vi "subsample_time_domain.vi"(8 "Array":cluster{"Array":dbl[]}[](array[cluster]), 10 "# sample points":i32, 11 "input array":dbl[][](array[numeric])) -> (3 "subsampled array":dbl[][](array[numeric]))   [LabVIEW 2016]
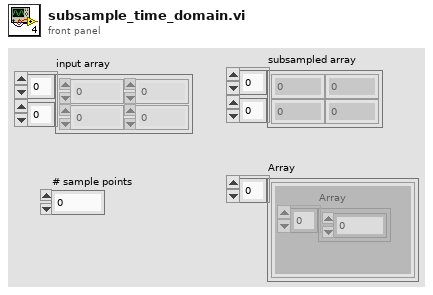
[diagram p1: front panel]
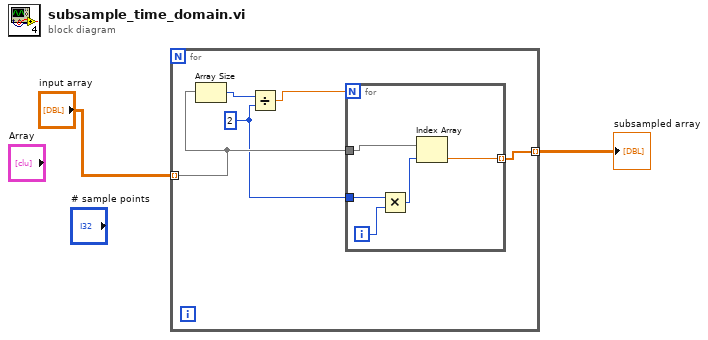
[diagram p0: block diagram]
diagram:
  n1 = for {
    tunnel: [w7] -> w2 mode=indexing
    tunnel: "input array" -> [w6] mode=indexing
    w3 = 2
    n2 = Array Size(array=w6) -> (size(s)=w5:i32)
    n3 = Divide(x=w5, y=w3) -> (x/y=w4:dbl)
    n4 = for {
      N: w4 -> [_]
      tunnel: w6 -> [w12]
      tunnel: [w10] -> w7 mode=indexing
      tunnel: w3 -> [w8]
      i -> [w9]
      n5 = Multiply(x=w8, y=w9) -> (x*y=w11:i32)
      n6 = Index Array(array=w12, index=w11) -> (element=w10:dbl)
    }
  }
  "subsampled array" <- w2
